vi "Station2_Data_Log.vi"(8 "error in (no error)":errorcluster, 9 "Station_QR":string, 11 "Cluster 2":T3) -> (0 "error out":errorcluster)   [LabVIEW 2017]
uses:
  <vilib>/addons/database/Connection.llb/Conn ObjectReference.ctl
  <vilib>/addons/database/NI_Database_API.lvlib
panel:
  in  "cluster":T1
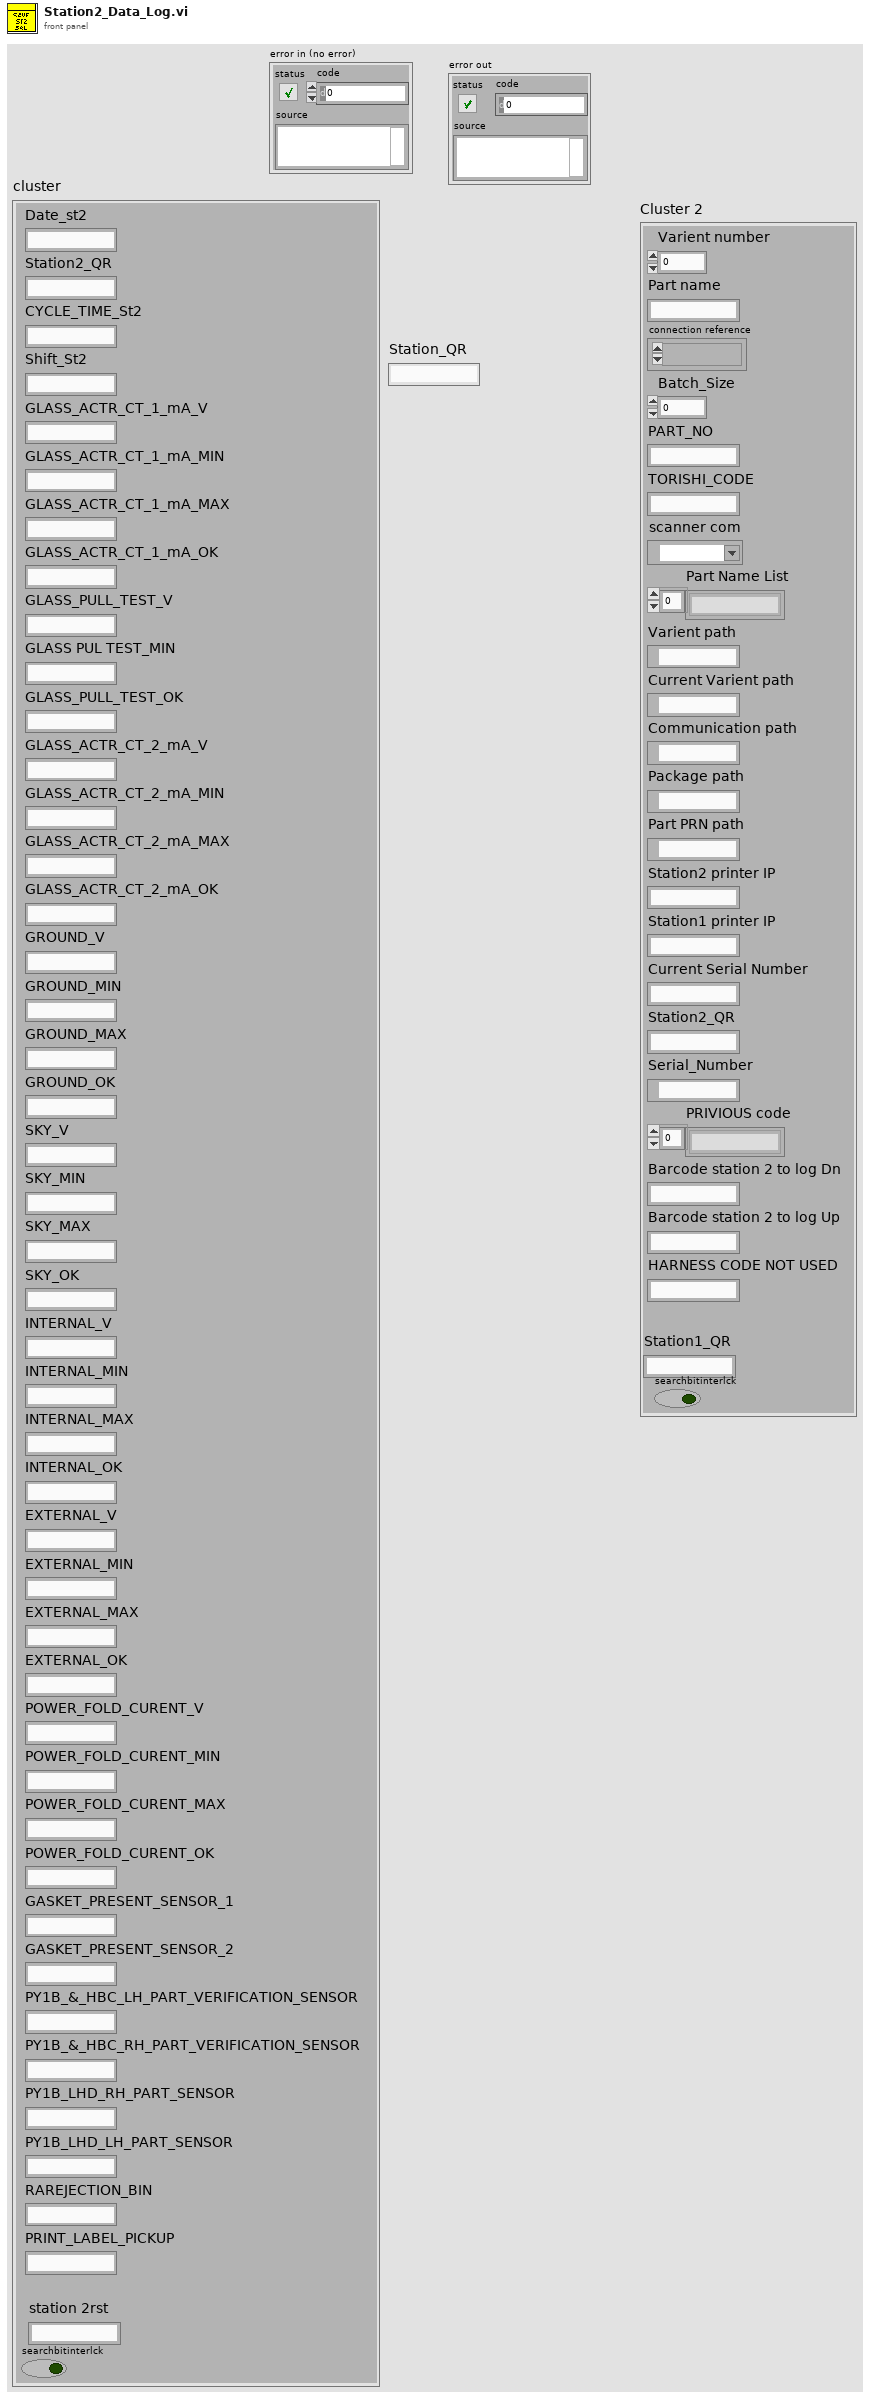
[diagram p1: front panel]
types:
  T1 = cluster{"columns[0]":string, "columns[1]":string, "columns[2]":string, "columns[3]":string, "columns[4]":string, "columns[5]":string, "columns[6]":string, "columns[7]":string, "columns[8]":string, "columns[9]":string, "columns[10]":string, "columns[11]":string, "columns[12]":string, "columns[13]":string, "columns[14]":string, "columns[15]":string, "columns[16]":string, "columns[17]":string, "columns[18]":string, "columns[19]":string, "columns[20]":string, "columns[21]":string, "columns[22]":string, "columns[23]":string, "columns[24]":string, "columns[25]":string, "columns[26]":string, "columns[27]":string, "columns[28]":string, "columns[29]":string, "columns[30]":string, "columns[31]":string, "columns[32]":string, "columns[33]":string, "columns[34]":string, "columns[35]":string, "columns[36]":string, "columns[37]":string, "columns[38]":string, "columns[39]":string, "columns[40]":string, "columns[41]":string, "columns[42]":string, "columns[42] 2":string, "searchbitinterlck":bool}
  T2 = typedef "NI_Database_API.lvlib/Conn ObjectReference.ctl" = refnum<k1>
  T3 = cluster{"Varient number":u16, "Part name":string, "connection reference":T2, "Batch_Size":u16, "PART_NO":string, "TORISHI_CODE":string, "scanner com":refnum<visa-resource-name>, "Part Name List":string[], "Varient path":path, "Current Varient path":path, "Communication path":path, "Package path":path, "Part PRN path":path, "Station2 printer IP":string, "Station1 printer IP":string, "Current Serial Number":string, "Station2_QR":string, "Serial_Number":path, "PRIVIOUS code":string[], "Barcode station 2 to log Dn":string, "Barcode station 2 to log Up":string, "HARNESS CODE NOT USED":string, "Station1_QR":string, "searchbitinterlck":bool}
  T4 = cluster{"columns[0]":string, "columns[1]":string, "columns[2]":string, "columns[3]":string, "columns[4]":string, "columns[5]":string, "columns[6]":string, "columns[7]":string, "columns[8]":string, "columns[9]":string, "columns[10]":string, "columns[11]":string, "columns[12]":string, "columns[13]":string, "columns[14]":string, "columns[15]":string, "columns[16]":string, "columns[17]":string, "columns[18]":string, "columns[19]":string, "columns[20]":string, "columns[21]":string, "columns[22]":string, "columns[23]":string, "columns[24]":string, "columns[25]":string, "columns[26]":string, "columns[27]":string, "columns[28]":string, "columns[29]":string, "columns[30]":string, "columns[31]":string, "columns[32]":string, "columns[33]":string, "columns[34]":string, "columns[35]":string, "columns[36]":string, "columns[37]":string, "columns[38]":string, "columns[39]":string, "columns[40]":string, "columns[41]":string, "columns[42]":string}
  T5 = typedef "LVDateTimeRec.ctl" = cluster{"fractional second":dbl, "second":i32, "minute":i32, "hour":i32, "day of month":i32, "month":i32, "year":i32, "day of week":i32, "day of year":i32, "DST":i32}
  T6 = cluster{"time stamp":timestamp, "Station2_QR":string, string, string, "Numeric 2":string, "Numeric 2":string, "Numeric 2":string, string, "Numeric 2":string, "Numeric 2":string, string, "Numeric 2":string, "Numeric 2":string, "Numeric 2":string, string, "Numeric 2":string, "Numeric 2":string, "Numeric 2":string, string, "Numeric 2":string, "Numeric 2":string, "Numeric 2":string, string, "Numeric 2":string, "Numeric 2":string, "Numeric 2":string, string, "Numeric 2":string, "Numeric 2":string, "Numeric 2":string, string, "Numeric 2":string, "Numeric 2":string, "Numeric 2":string, string, string, string, string, string, string, string, string, string, string}
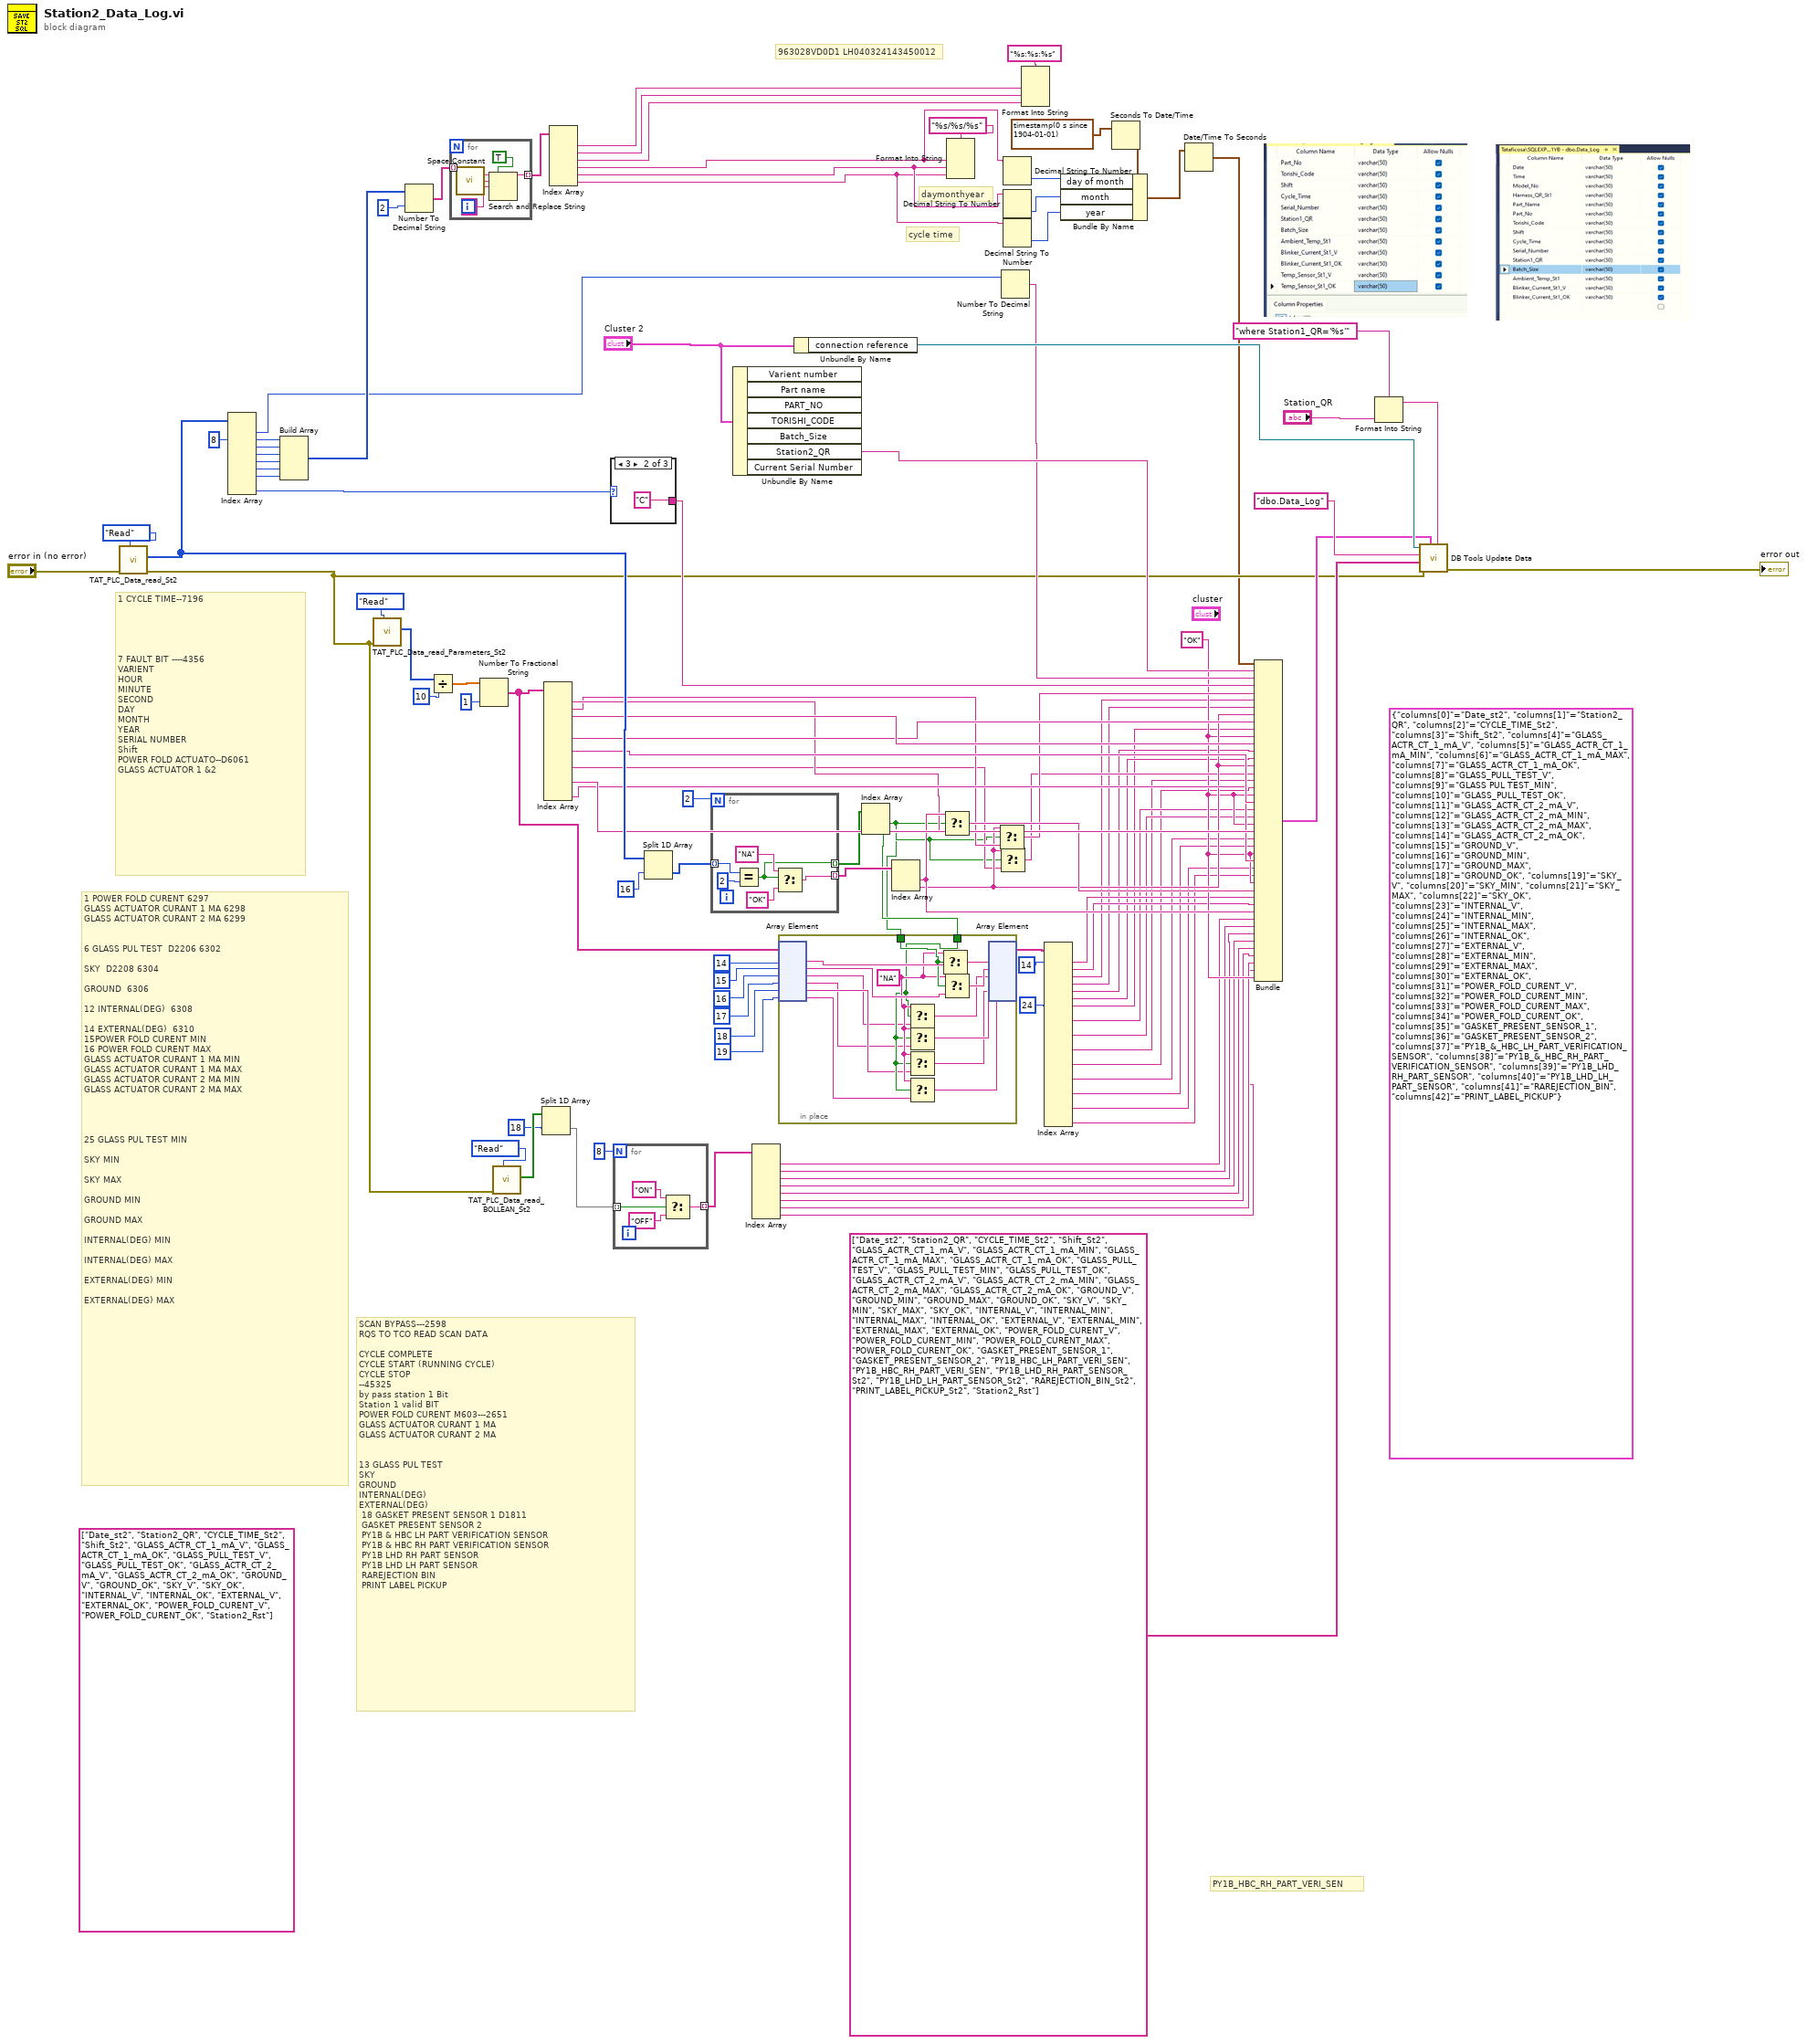
[diagram p0: block diagram]
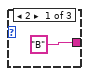
[diagram p2: hidden frame]
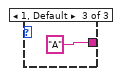
[diagram p3: hidden frame]
diagram:
  (unwired) T4 {"columns[0]"="Date_st2", "columns[1]"="Station2_QR", "columns[2]"="CYCLE_TIME_St2", "columns[3]"="Shift_St2", "columns[4]"="GLASS_ACTR_CT_1_mA_V", "columns[5]"="GLASS_ACTR_CT_1_mA_MIN", "columns[6]"="GLASS_ACTR_CT_1_mA_MAX", "columns[7]"="GLASS_ACTR_CT_1_mA_OK", "columns[8]"="GLASS_PULL_TEST_V", "columns[9]"="GLASS PUL TEST_MIN", "columns[10]"="GLASS_PULL_TEST_OK", "columns[11]"="GLASS_ACTR_CT_2_mA_V", "columns[12]"="GLASS_ACTR_CT_2_mA_MIN", "columns[13]"="GLASS_ACTR_CT_2_mA_MAX", "columns[14]"="GLASS_ACTR_CT_2_mA_OK", "columns[15]"="GROUND_V", "columns[16]"="GROUND_MIN", "columns[17]"="GROUND_MAX", "columns[18]"="GROUND_OK", "columns[19]"="SKY_V", "columns[20]"="SKY_MIN", "columns[21]"="SKY_MAX", "columns[22]"="SKY_OK", "columns[23]"="INTERNAL_V", "columns[24]"="INTERNAL_MIN", "columns[25]"="INTERNAL_MAX", "columns[26]"="INTERNAL_OK", "columns[27]"="EXTERNAL_V", "columns[28]"="EXTERNAL_MIN", "columns[29]"="EXTERNAL_MAX", "columns[30]"="EXTERNAL_OK", "columns[31]"="POWER_FOLD_CURENT_V", "columns[32]"="POWER_FOLD_CURENT_MIN", "columns[33]"="POWER_FOLD_CURENT_MAX", "columns[34]"="POWER_FOLD_CURENT_OK", "columns[35]"="GASKET_PRESENT_SENSOR_1", "columns[36]"="GASKET_PRESENT_SENSOR_2", "columns[37]"="PY1B_&_HBC_LH_PART_VERIFICATION_SENSOR", "columns[38]"="PY1B_&_HBC_RH_PART_VERIFICATION_SENSOR", "columns[39]"="PY1B_LHD_RH_PART_SENSOR", "columns[40]"="PY1B_LHD_LH_PART_SENSOR", "columns[41]"="RAREJECTION_BIN", "columns[42]"="PRINT_LABEL_PICKUP"} ("cluster 2")
  (unwired) string[] ["Date_st2", "Station2_QR", "CYCLE_TIME_St2", "Shift_St2", "GLASS_ACTR_CT_1_mA_V", "GLASS_ACTR_CT_1_mA_OK", "GLASS_PULL_TEST_V", "GLASS_PULL_TEST_OK", "GLASS_ACTR_CT_2_mA_V", "GLASS_ACTR_CT_2_mA_OK", "GROUND_V", "GROUND_OK", "SKY_V", "SKY_OK", "INTERNAL_V", "INTERNAL_OK", "EXTERNAL_V", "EXTERNAL_OK", "POWER_FOLD_CURENT_V", "POWER_FOLD_CURENT_OK", "Station2_Rst"] ("columns")
  w54 = "OK"
  # "PY1B_HBC_RH_PART_VERI_SEN"
  # "SCAN BYPASS---2598\nRQS TO TCO READ SCAN DATA \n\nCYCLE COMPLETE\nCYCLE START (RUNNING CYCLE)\nCYCLE STOP\n--45325\nby pass station 1 Bit\nStation 1 valid BIT\nPOWER FOLD CURENT M603---2651\nGLASS ACTUATOR CURANT 1 MA\nGLASS ACTUATOR CURANT 2 MA\n\n\n13 GLASS PUL TEST\nSKY \nGROUND\nINTERNAL(DEG)\nEXTERNAL(DEG)\n 18 GASKET PRESENT SENSOR 1 D1811\n GASKET PRESENT SENSOR 2\n PY1B & HBC LH PART VERIFICATION SENSOR\n PY1B & HBC RH PART VERIFICATION SENSOR\n PY1B LHD RH PART SENSOR\n PY1B LHD LH PART SENSOR\n RAREJECTION BIN\n PRINT LABEL PICKUP"
  # "1 POWER FOLD CURENT 6297\nGLASS ACTUATOR CURANT 1 MA 6298\nGLASS ACTUATOR CURANT 2 MA 6299\n\n\n6 GLASS PUL TEST  D2206 6302\n\nSKY  D2208 6304\n\nGROUND  6306\n\n12 INTERNAL(DEG)  6308\n\n14 EXTERNAL(DEG)  6310\n15POWER FOLD CURENT MIN\n16 POWER FOLD CURENT MAX\nGLASS ACTUATOR CURANT 1 MA MIN\nGLASS ACTUATOR CURANT 1 MA MAX\nGLASS ACTUATOR CURANT 2 MA MIN\nGLASS ACTUATOR CURANT 2 MA MAX\n\n\n\n\n25 GLASS PUL TEST MIN\n\nSKY MIN\n\nSKY MAX\n\nGROUND MIN\n\nGROUND MAX\n\nINTERNAL(DEG) MIN\n\nINTERNAL(DEG) MAX\n\nEXTERNAL(DEG) MIN\n\nEXTERNAL(DEG) MAX"
  # "1 CYCLE TIME--7196\n\n\n\n\n\n7 FAULT BIT ----4356\nVARIENT\nHOUR\nMINUTE\nSECOND\nDAY\nMONTH\nYEAR\nSERIAL NUMBER\nShift\nPOWER FOLD ACTUATO--D6061\nGLASS ACTUATOR 1 &2"
  # "daymonthyear"
  # "963028VD0D1 LH040324143450012"
  # "cycle time"
  n1 = call "TAT_PLC_Data_read_St2.vi"("Enum"=enum16{"Read", "Write"}."Read", "error in (no error)"="error in (no error)") -> ("error out"=w24:errorcluster, "Array 2"=w77:u16[])  [unwired: 8 in]
  n2 = Index Array(array=w77, index #2=8 ("index")) -> (element #1=w86:u16, element #2=w103:u16, element #3=w102:u16, element #4=w101:u16, element #5=w100:u16, element #6=w99:u16, element #7=w98:u16, element #9=w91:u16)  [unwired: 8 in, 1 out]
  n3 = Build Array(w103, w102, w101, w100, w99, w98) -> (w97:u16[])
  n4 = call "TAT_PLC_Data_read_Parameters_St2.vi"("Enum"=enum16{"Read", "Write"}."Read", "error in (no error)"=w24) -> ("Array 2"=w70:u16[])  [unwired: 8 in, 1 out]
  n5 = Number To Decimal String(number=w97, width (-)=i16 2) -> (decimal integer string=w106:string[])
  n6 = Divide(x=w70, y=10 ("Numeric 2")) -> (x/y=w72:dbl[])
  n7 = for {
    tunnel: w106 -> [w111] mode=indexing
    tunnel: [w110] -> w105 mode=indexing
    n8 = call <vilib>:"Space Constant.vi"() -> ("String"=w112:string)
    n9 = Search and Replace String(replace all?=TRUE ("replace all? (F)"), input string=w111, search string=w112, replace string="0" ("replace string (\"\")")) -> (result string=w110:string)  [unwired: 4 in, 3 out]
  }
  n10 = Number To Fractional String(number=w72, precision (6)=i16 1) -> (F-format string=w52:string[])  [unwired: 2 in]
  n11 = call "TAT_PLC_Data_read_BOLLEAN_St2.vi"("Enum"=enum16{"Read", "Write"}."Read", "error in (no error)"=w24) -> ("Array 2"=w23:bool[])  [unwired: 8 in, 1 out]
  n12 = Split 1D Array(array=w23, index=18) -> (second subarray=w21:bool[])  [unwired: 1 out]
  n13 = Index Array(array=w52) -> (element #1=w63:string, element #2=w61:string, element #3=w69:string, element #6=w68:string, element #8=w67:string, element #10=w58:string, element #12=w66:string, element #14=w65:string)  [unwired: 14 in, 6 out]
  n14 = Index Array(array=w105) -> (element #1=w95:string, element #2=w94:string, element #3=w93:string, element #4=w1:string, element #5=w5:string, element #6=w4:string)  [unwired: 6 in]
  n15 = case shown="3" w91 {
    tunnel: ["B" "C" "A"] -> w75
    frame 2 {
    }
    frame 3 {
    }
    frame 1, Default {
    }
  }
  n16 = for {
    N: 8 -> [_]
    tunnel: w21 -> [w119] mode=indexing
    tunnel: [w118] -> w19 mode=indexing
    n17 = Select(t="ON", s=w119, f="OFF") -> (s? t:f=w118:string)
  }
  n18 = Split 1D Array(array=w77, index=16) -> (second subarray=w89:u16[])  [unwired: 1 out]
  n19 = for {
    N: 2 -> [_]
    tunnel: w89 -> [w127] mode=indexing
    tunnel: [w123] -> w87 mode=indexing
    tunnel: [w122] -> w49 mode=indexing
    n20 = Equal?(x=w127, y=2) -> (x = y?=w122:bool)
    n21 = Select(t="NA", s=w122, f="OK") -> (s? t:f=w123:string)
  }
  n22 = Unbundle By Name("Cluster 2") -> ("Station2_QR"=w76:string)  [unwired: 6 out]
  n23 = Index Array(array=w19) -> (element #1=w18:string, element #2=w17:string, element #3=w16:string, element #4=w15:string, element #5=w14:string, element #6=w13:string, element #7=w12:string, element #8=w11:string)  [unwired: 8 in]
  n24 = Unbundle By Name("Cluster 2") -> ("connection reference"=w83:T2)
  n25 = Index Array(array=w49) -> (element #1=w47:bool, element #2=w48:bool)  [unwired: 2 in]
  n26 = in-place {
    in-place-border: w48 -> [w136]
    in-place-border: w47 -> [w138]
    w137 = "NA"
    n27 = in-place-array #1(w52, 14 ("index"), 15 ("index"), 16 ("index"), 17 ("index"), 18 ("index"), 19 ("index")) -> (w142:string, w139:string, w132:string, w133:string, w134:string, w135:string)
    n28 = Select(t=w137, s=w136, f=w132) -> (s? t:f=w131:string)
    n29 = Select(t=w137, s=w136, f=w133) -> (s? t:f=w130:string)
    n30 = Select(t=w137, s=w136, f=w134) -> (s? t:f=w129:string)
    n31 = Select(t=w137, s=w136, f=w135) -> (s? t:f=w128:string)
    n32 = Select(t=w137, s=w138, f=w142) -> (s? t:f=w141:string)
    n33 = Select(t=w137, s=w138, f=w139) -> (s? t:f=w140:string)
    n34 = in-place-array #1(w141, w140, w131, w130, w129, w128) -> (w42:string[])  [unwired: 6 out]
  }
  n35 = Index Array(array=w87) -> (element #1=w64:string, element #2=w59:string)  [unwired: 2 in]
  n36 = Select(t=w64, s=w47, f=w63) -> (s? t:f=w62:string)
  n37 = Format Into String(format string="%s/%s/%s" ("time format string (%c)"), w1, w5, w4) -> ()  [unwired: 2 in, 2 out]
  n38 = Select(t=w59, s=w48, f=w61) -> (s? t:f=w60:string)
  n39 = Select(t=w59, s=w48, f=w58) -> (s? t:f=w57:string)
  n40 = Number To Decimal String(number=w86) -> (decimal integer string=w56:string)  [unwired: 1 in]
  n41 = Decimal String To Number(string=w1) -> (number=w8:i32)  [unwired: 2 in, 1 out]
  n42 = Decimal String To Number(string=w5) -> (number=w7:i32)  [unwired: 2 in, 1 out]
  n43 = Decimal String To Number(string=w4) -> (number=w6:i32)  [unwired: 2 in, 1 out]
  n44 = Format Into String(format string="%s:%s:%s" ("time format string (%c)"), w95, w94, w93) -> ()  [unwired: 2 in, 2 out]
  n45 = Index Array(array=w42, index #1=14 ("index"), index #7=24 ("index")) -> (element #1=w40:string, element #2=w39:string, element #3=w38:string, element #4=w37:string, element #5=w36:string, element #6=w35:string, element #7=w34:string, element #9=w33:string, element #11=w32:string, element #13=w31:string, element #15=w30:string, element #17=w29:string, element #19=w28:string, element #21=w27:string, element #23=w26:string)  [unwired: 21 in, 8 out]
  n46 = Seconds To Date/Time(time stamp (now)=timestamp(0 s since 1904-01-01)) -> (date time rec=w10:T5)  [unwired: 1 in]
  n47 = Bundle By Name(cluster=w10, "day of month"=w8, "month"=w7, "year"=w6) -> (w9:T5)
  n48 = Date/Time To Seconds(2:w9) -> (0:w2:timestamp)  [unwired: 1 in]
  n49 = Bundle("time stamp"=w2, "Station2_QR"=w76, w56, w75, "Numeric 2"=w60, "Numeric 2"=w38, "Numeric 2"=w37, w59, "Numeric 2"=w68, "Numeric 2"=w34, w54, "Numeric 2"=w69, "Numeric 2"=w36, "Numeric 2"=w35, w59, "Numeric 2"=w57, "Numeric 2"=w31, "Numeric 2"=w30, w54, "Numeric 2"=w67, "Numeric 2"=w33, "Numeric 2"=w32, w54, "Numeric 2"=w66, "Numeric 2"=w29, "Numeric 2"=w28, w54, "Numeric 2"=w65, "Numeric 2"=w27, "Numeric 2"=w26, w54, "Numeric 2"=w62, "Numeric 2"=w40, "Numeric 2"=w39, w64, w18, w17, w16, w15, w14, w13, w12, w11, w54) -> (w55:T6)  [unwired: 1 in]
  n50 = Format Into String(format string="where Station1_QR='%s'", "Station_QR") -> (resulting string=w78:string)  [unwired: 2 in, 1 out]
  n51 = call <vilib>:"DB Tools Update Data.vi"("condition"=w78, "data"=w55, "error in (no error)"=w24, "columns"=string[] ["Date_st2", "Station2_QR", "CYCLE_TIME_St2", "Shift_St2", "GLASS_ACTR_CT_1_mA_V", "GLASS_ACTR_CT_1_mA_MIN", "GLASS_ACTR_CT_1_mA_MAX", "GLASS_ACTR_CT_1_mA_OK", "GLASS_PULL_TEST_V", "GLASS_PULL_TEST_MIN", "GLASS_PULL_TEST_OK", "GLASS_ACTR_CT_2_mA_V", "GLASS_ACTR_CT_2_mA_MIN", "GLASS_ACTR_CT_2_mA_MAX", "GLASS_ACTR_CT_2_mA_OK", "GROUND_V", "GROUND_MIN", "GROUND_MAX", "GROUND_OK", "SKY_V", "SKY_MIN", "SKY_MAX", "SKY_OK", "INTERNAL_V", "INTERNAL_MIN", "INTERNAL_MAX", "INTERNAL_OK", "EXTERNAL_V", "EXTERNAL_MIN", "EXTERNAL_MAX", "EXTERNAL_OK", "POWER_FOLD_CURENT_V", "POWER_FOLD_CURENT_MIN", "POWER_FOLD_CURENT_MAX", "POWER_FOLD_CURENT_OK", "GASKET_PRESENT_SENSOR_1", "GASKET_PRESENT_SENSOR_2", "PY1B_HBC_LH_PART_VERI_SEN", "PY1B_HBC_RH_PART_VERI_SEN", "PY1B_LHD_RH_PART_SENSOR_St2", "PY1B_LHD_LH_PART_SENSOR_St2", "RAREJECTION_BIN_St2", "PRINT_LABEL_PICKUP_St2", "Station2_Rst"], "table"="dbo.Data_Log", "connection reference"=w83) -> ("error out"=→"error out":errorcluster)  [unwired: 4 in, 1 out]
